vi "Run Test - Parameter Calculation (SubVI).vi"(6 "Tab Control":T2, 7 "DS in":T3 {"M Event" items=["Stop", "Running", "PID", "Up Limit", "Down Limit", "Load Limit"]; "Test Type" items=["Please Select", "Triaxial Shear", "Triaxial UU", "Shearbox", "Permeability", "Consolidation (Stepped Loading)/Swelling", "Saturation (Incremental)", "User Defined", "UCT", "Isotropic Consolidation", "Swelling Pressure"]; "Data"."Test Type" items=["Please Select", "Triaxial Shear", "Triaxial UU", "Shearbox", "Permeability", "Consolidation (Stepped Loading)/Swelling", "Saturation (Incremental)", "User Defined", "UCT", "Isotropic Consolidation", "Swelling Pressure"]}, 8 "error in (no error)":errorcluster, 9 "Decimal In":u8[](array[numeric]), 10 "Log Data In":string[](array[string]), 11 "Sensor Data In":sgl[](array[numeric])) -> (0 "error out":errorcluster, 3 "output cluster":T1, 5 "DS out":T3 {"M Event" items=["Stop", "Running", "PID", "Up Limit", "Down Limit", "Load Limit"]; "Test Type" items=["Please Select", "Triaxial Shear", "Triaxial UU", "Shearbox", "Permeability", "Consolidation (Stepped Loading)/Swelling", "Saturation (Incremental)", "User Defined", "UCT", "Isotropic Consolidation", "Swelling Pressure"]; "Data"."Test Type" items=["Please Select", "Triaxial Shear", "Triaxial UU", "Shearbox", "Permeability", "Consolidation (Stepped Loading)/Swelling", "Saturation (Incremental)", "User Defined", "UCT", "Isotropic Consolidation", "Swelling Pressure"]})   [LabVIEW 2019]
uses:
  Controls/RunTest - Data Structure.ctl
  Controls/Test Panel - Data Structure.ctl
  Controls/Station - Test Type.ctl
  <vilib>/Utility/miscctls.llb/LVRowAndColumnTypeDef.ctl
  Controls/RunTest - Calculate Data.ctl
  <vilib>/httpClient/ClientHandle.ctl
  Controls/RunTest - Start Condition.ctl
  Controls/RunTest - Stop Condition.ctl
  Controls/UDP - Event.ctl
  Controls/RunTest - Tab Test Type.ctl
  <vilib>/httpClient/LabVIEWHTTPClient.lvlib
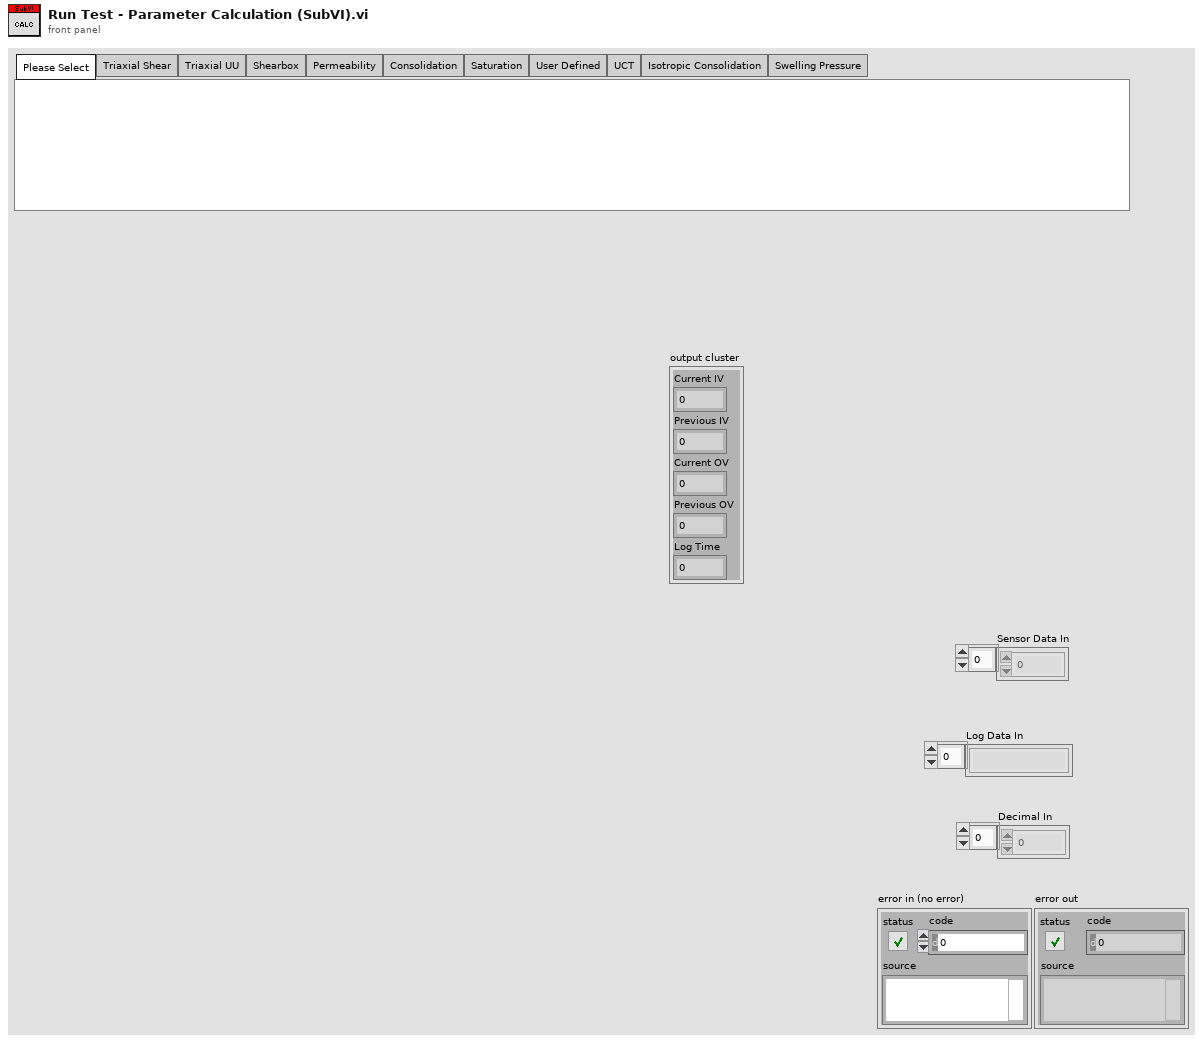
[diagram p1: front panel]
types:
  T1 = cluster{"Current IV":dbl, "Previous IV":dbl, "Current OV":dbl, "Previous OV":dbl, "Log Time":dbl}
  T2 = typedef "RunTest - Tab Test Type.ctl" = enum32{"Please Select", "Triaxial Shear", "Triaxial UU", "Shearbox", "Permeability", "Consolidation", "Saturation", "User Defined", "UCT", "Isotropic Consolidation", "Swelling Pressure"}
  T3 = typedef "RunTest - Data Structure.ctl" = cluster{"Test Plan":string[], "PlanRow":i32, "Device Name":string[], "Timeout":i32, "Start?":bool, "Pause?":bool, "IP Address":string[], "LogRow":i32, "Logtype":u16, "Log Elapse":sgl, "Data":T4, "Stop log?":bool, "tdms":refnum<k34>, "Sensor Data":sgl[], "Start time":timestamp, "Prev Log Elapse":u32, "Plot":u16, "X-Axis":u16[], "Y-Axis":u16[], "XY":cluster{"X":dbl, "Y":dbl}[][], "End Stage?":bool, "1run":bool, "Condition":u16[], "Start Con":bool, "Log Con":bool, "Stop Con":bool, "Start Elapse":dbl, "Start Load":dbl, "Motor":i32, "StartRow":i32, "number log":i32, "Dir":bool, "Start time test":timestamp, "Auto":bool, "Check return?":bool, "Inv":cluster{"M":i32[], "Bool":bool[]}, "tdms temp":refnum<k34>, "Zero?":bool, "Plot Timer":dbl, "1st Run":bool, "TDMS Path":path, "MaxLoad":dbl, "Log Timer":sgl[], "Test Type":T5, "Log Sensor":string[], "Save?":bool, "1st Log":bool, "Y-Axis 2":u16[], "On Y-Axis 2":bool, "Decimal":u8[], "Init":cluster{"PWP TS":sgl, "Load TS":sgl, "Volume TS":sgl, "Disp TS":sgl, "CP":sgl, "Vol In":sgl, "Vol Out":sgl, "Load UCT":sgl, "Disp UCT":sgl, "PWP Sat":sgl, "CP Sat":sgl, "Volume IsoCons":sgl, "PWP IsoCons":sgl, "PWP TUU":sgl, "Load TUU":sgl, "Volume TUU":sgl, "Disp TUU":sgl, "Load Cons":sgl, "Disp Cons":sgl, "Volume Sat":sgl, "Vertical Load SB":sgl, "Vertical Disp SB":sgl, "H Disp SB":sgl, "H Load SB":sgl}, "Calc":T7, "Device Index":i32[], "Channel Index":i32[], "http ref":T8, "fileid":string, "Step Cons":cluster{"V Stress":sgl, "H Settlement":sgl}, "RunTest":bool, "Graph Last":i32, "Init?":bool, "Datalog":bool[], "Start":T9, "Stop":T10, "Running?":bool, "StartTime":dbl, "Log Prev Time":dbl, "KeyName":string[], "Test RunTime":dbl, "Log Prev Axial":dbl, "M Event":T11[], "Last Log":bool, "popup":bool, "PreStart UU":bool, "PreStart Sat":bool}
  T4 = typedef "Test Panel - Data Structure.ctl" = cluster{"Station":string, "Sample ID":string, "Job No":string, "Job Description":string, "Filename":string, "Test Type":T5, "Speciment No":string, "Depth":string, "Height":string, "Diameter/Length":string, "Weight":string, "Test Parameter":string, "Station[]":string[], "Edit Pos":T6, "Edit Pos Prev":T6, "Area":string, "Path":string}
  T5 = typedef "Station - Test Type.ctl" = u16
  T6 = typedef "LVRowAndColumnTypeDef.ctl" = cluster{"Row":i32, "Column":i32}
  T7 = typedef "RunTest - Calculate Data.ctl" = cluster{"TS":cluster{"Change PWP":sgl, "Change Vol":sgl, "Axial Load":sgl, "CiL":sgl, "Deviator":sgl, "Axial Strain":sgl, "MaxDeviator":sgl}, "TUU":cluster{"Change PWP":sgl, "Axial Load":sgl, "CiL":sgl, "Deviator":sgl, "Axial Strain":sgl, "MaxDeviator":sgl}, "Sat":cluster{"B Value":sgl, "PWP Diss":sgl, "CPP":sgl, "CV":sgl}, "Per":cluster{"Change Vol In":sgl, "Change Vol Out":sgl, "Mean Vol":sgl, "Gradient Pressure":sgl, "Outlet Flow":sgl, "Inlet Flow":sgl, "I X1":sgl, "I X2":sgl, "I Y1":sgl, "I Y2":sgl, "O X1":sgl, "O X2":sgl, "O Y1":sgl, "O Y2":sgl}, "Step Cons":cluster{"V Stress":sgl, "H Settlement":sgl, "Total H Settle":sgl, "Prev Total H":sgl}, "UCT":cluster{"ALC":sgl, "H Change":sgl, "Deviator":sgl, "Axial Strain":sgl, "V Stress":sgl, "MaxDeviator":sgl}, "ISO Cons":cluster{"CPP":sgl, "PWP Diss":sgl, "CV":sgl}, "SB":cluster{"Speci LenC":sgl, "Shear Strain":sgl, "H LC":sgl, "Normal Stress":sgl, "Shear Stress":sgl, "MaxShear":sgl}}
  T8 = typedef "LabVIEWHTTPClient.lvlib/ClientHandle.ctl" = refnum<k1>
  T9 = typedef "RunTest - Start Condition.ctl" = cluster{"Cons":cluster{"VS":dbl, "Delay":bool, "No Delay":dbl}, "Sat":cluster{"CP":dbl, "BP":dbl, "StartBP":bool, "Target CP":bool, "Target BP":bool}, "Iso":cluster{"Select":dbl, "BP":dbl, "IC2":dbl, "IC3":dbl, "IC4":dbl, ". IC6":bool, "IC6":dbl, "IC6-2":dbl, "Target":bool, "Time Cond":dbl, "Last PWP":dbl}, "TS":cluster{"SS":dbl, "Engage":bool, "ES":dbl, "LC":dbl, "PreStart":bool, "Trig SS":bool, "Drain":dbl}, "TUU":cluster{"SS":dbl, "Engage":bool, "ES":dbl, "LC":dbl, "PreStart":bool, "Trig SS":bool, "CP":dbl, "Delay Value":dbl, "Delay":bool, "CP PID":bool}, "UCT":cluster{"SS":dbl, "Engage":bool, "ES":dbl, "LC":dbl, "PreStart":bool, "Trig SS":bool}, "Enable?":bool, "SB":cluster{"SS":dbl, "Engage":bool, "ES":dbl, "LC":dbl, "PreStart":bool, "Trig SS":bool, "VS":dbl, "Delay Value":dbl, "Delay":bool, "VS PID":bool}, "Perm":cluster{"DP":dbl}}
  T10 = typedef "RunTest - Stop Condition.ctl" = cluster{"Cons":cluster{"Select":i32, "Disp":dbl, "Time":dbl, "Time2":dbl, "Disp 2":dbl, "Time Cond":dbl, "Last Disp":dbl, "Swell":bool}, "Sat":cluster{"Select":i32, "PP":dbl, "Time":dbl, "VC":dbl, "Time2":dbl, "Time Cond":dbl, "Last PP":dbl, ".B":bool, "B":dbl, "Last Vc":dbl, "Time Cond 2":dbl, "Time3":dbl, "Time Cond 3":dbl, "B Achieve":bool}, "Iso":cluster{"PP":dbl, "Time":dbl, "VC":dbl, "Time2":dbl, "Time Cond":dbl, "Last Vc":dbl, ".PP":bool, "Time Cond 2":dbl, "Select":i32}, "TS":cluster{"Axial":dbl, ".MaxDev":bool, "MaxDev Value":dbl, "Return":bool, "Reset":bool, "Prev Time":dbl, "PostStop Run":bool, "CP Stop":bool, "BP Stop":bool, "PostStop Trig":bool, "Reset Value":dbl, "BPTrig":bool, "CPTrig":bool, "VLCTrig":bool}, "TUU":cluster{"Axial":dbl, ".MaxDev":bool, "MaxDev Value":dbl, "Return":bool, "Reset":bool, "Prev Time":dbl, "PostStop Run":bool, "CP Stop":bool, "BP Stop":bool, "PostStop Trig":bool, "Reset Value":dbl, "BPTrig":bool, "CPTrig":bool, "VLCTrig":bool}, "UCT":cluster{"Axial":dbl, ".MaxDev":bool, "MaxDev Value":dbl, "Return":bool, "Reset":bool, "Prev Time":dbl, "PostStop Run":bool, "CP Stop":bool, "BP Stop":bool, "PostStop Trig":bool}, "Enable?":bool, "SB":cluster{"Shear":dbl, ".MaxShear":bool, "MaxShear Value":dbl, "Return":bool, "Reset":bool, "Prev Time":dbl, "PostStop Run":bool, "CP Stop":bool, "BP Stop":bool, "PostStop Trig":bool, "Reset Value":dbl, "BPTrig":bool, "CPTrig":bool, "VLCTrig":bool}, "Perm":cluster{"Max Time":bool, "Reset":bool, "PostStop Run":bool, "Ratio":bool, "Reset Value":dbl, "Time":dbl, "RatioTime":dbl, "RatioMore":dbl, "RatioLess":dbl, "Time Cond":dbl, "Time Cond 2":dbl, "Prev IF":dbl, "Prev OF":dbl, "PostStop Trig":bool, "BP Trig":bool, "DP Stop":bool, "BP Stop":bool, "CP Stop":bool, "CP Trig":bool}, "SP":cluster{".Max Time":bool, ".Time":bool, "Time":dbl, "MaxTime":dbl, "Time Cond":dbl, "Max Time Cond":dbl, "Stress":dbl}}
  T11 = typedef "UDP - Event.ctl" = u16
  T12 = cluster{"Current IV":dbl, "Previous IV":dbl, "Current OV":dbl, "Previous OV":dbl, "Log time":dbl}
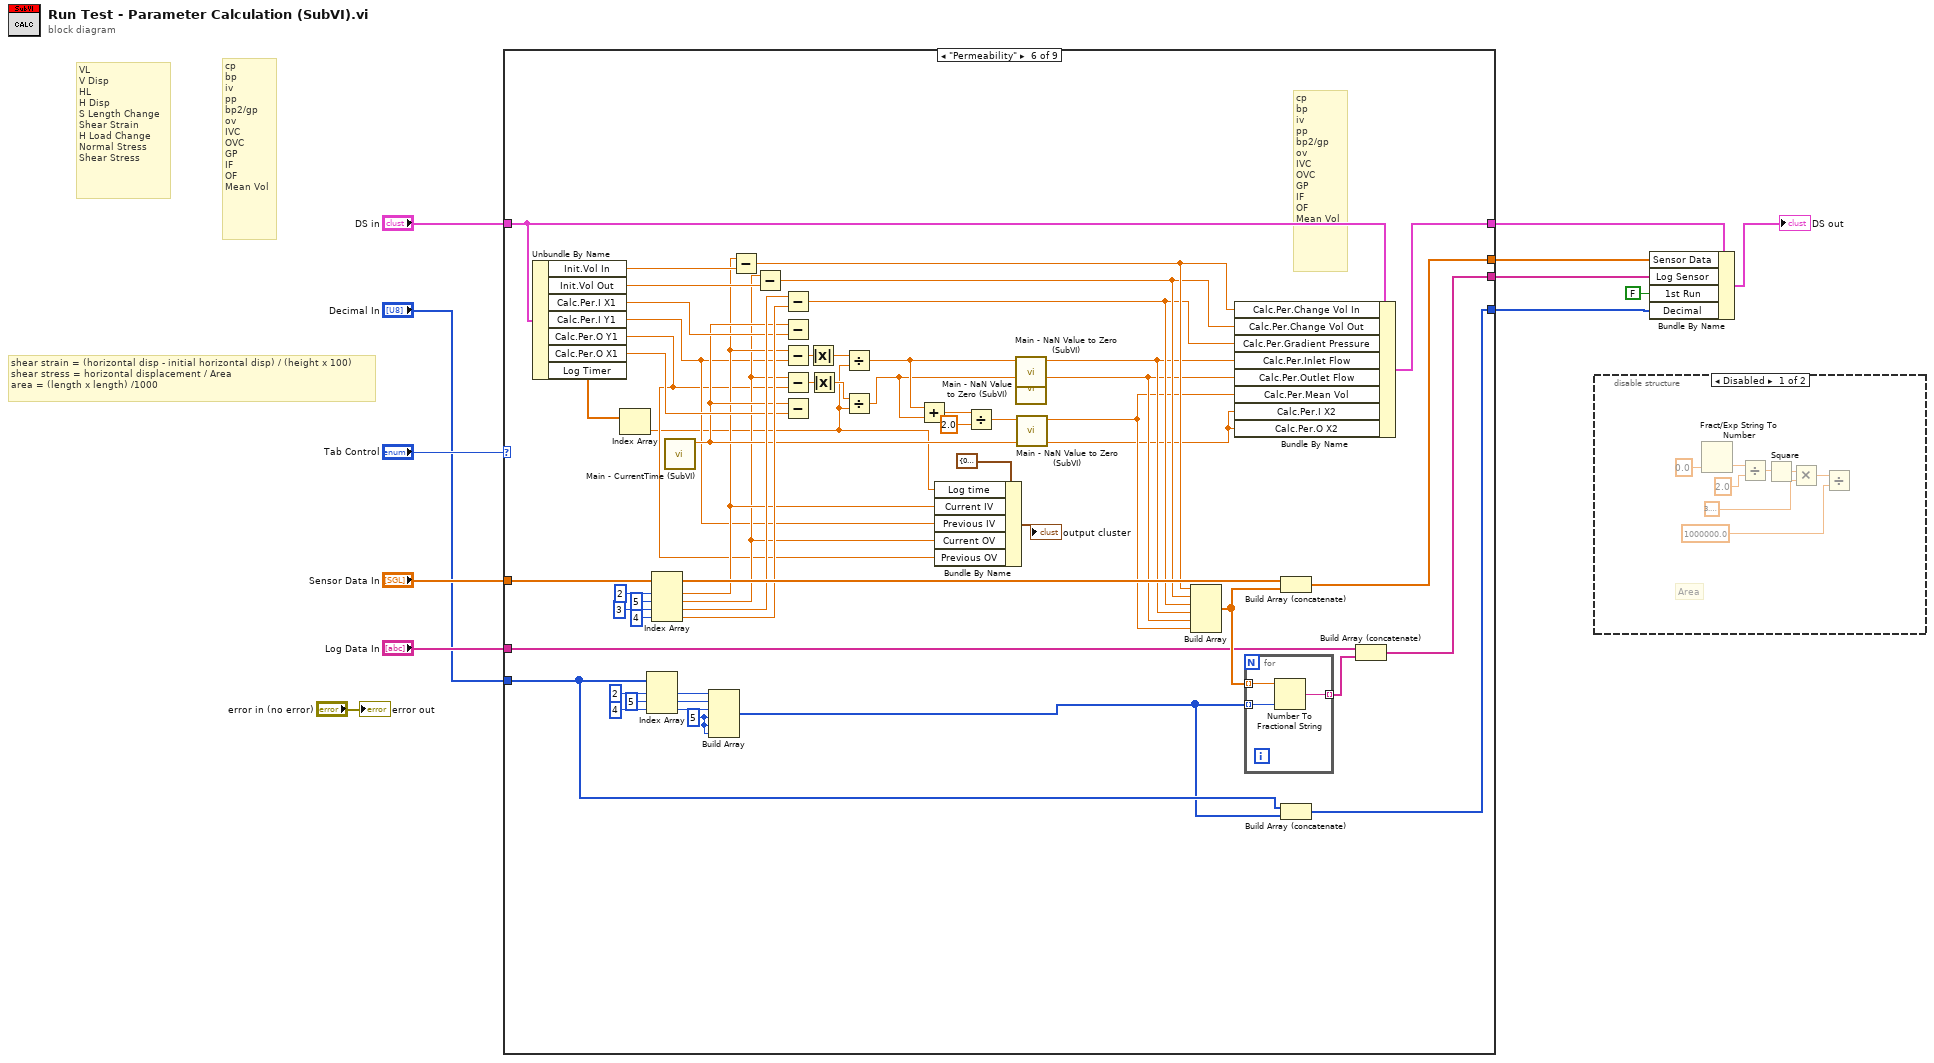
[diagram p0: block diagram]
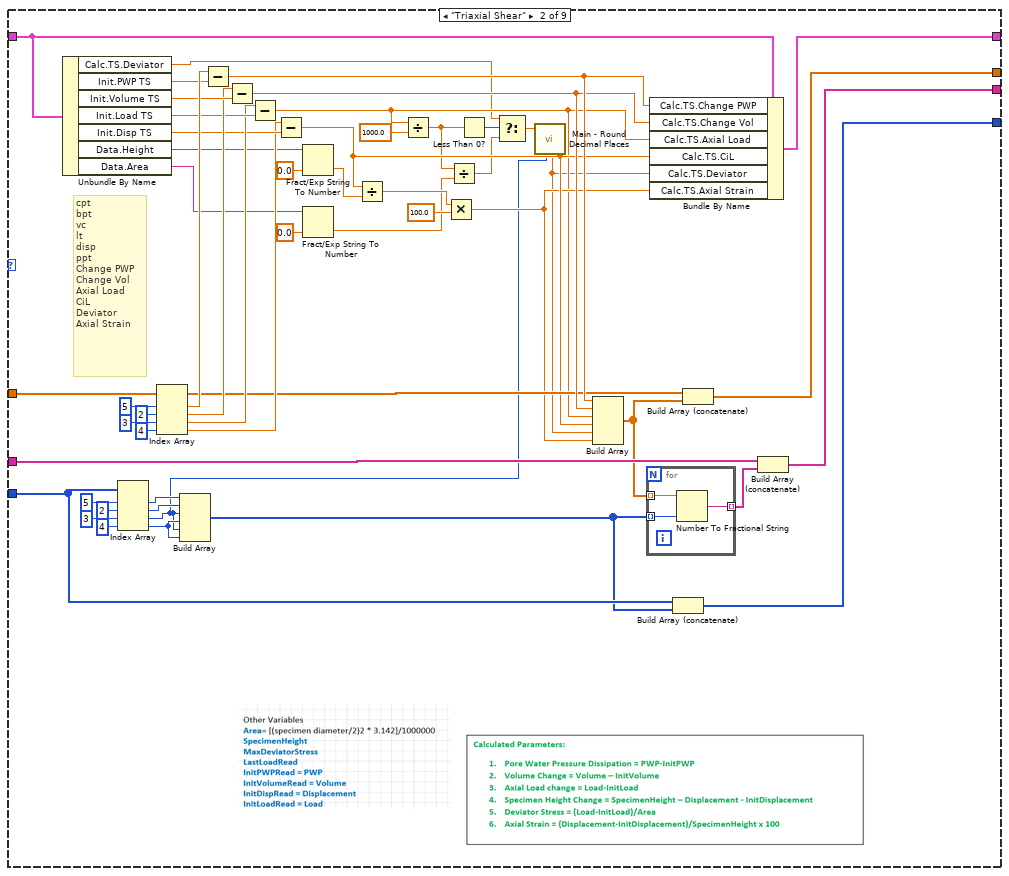
[diagram p4: hidden frame]
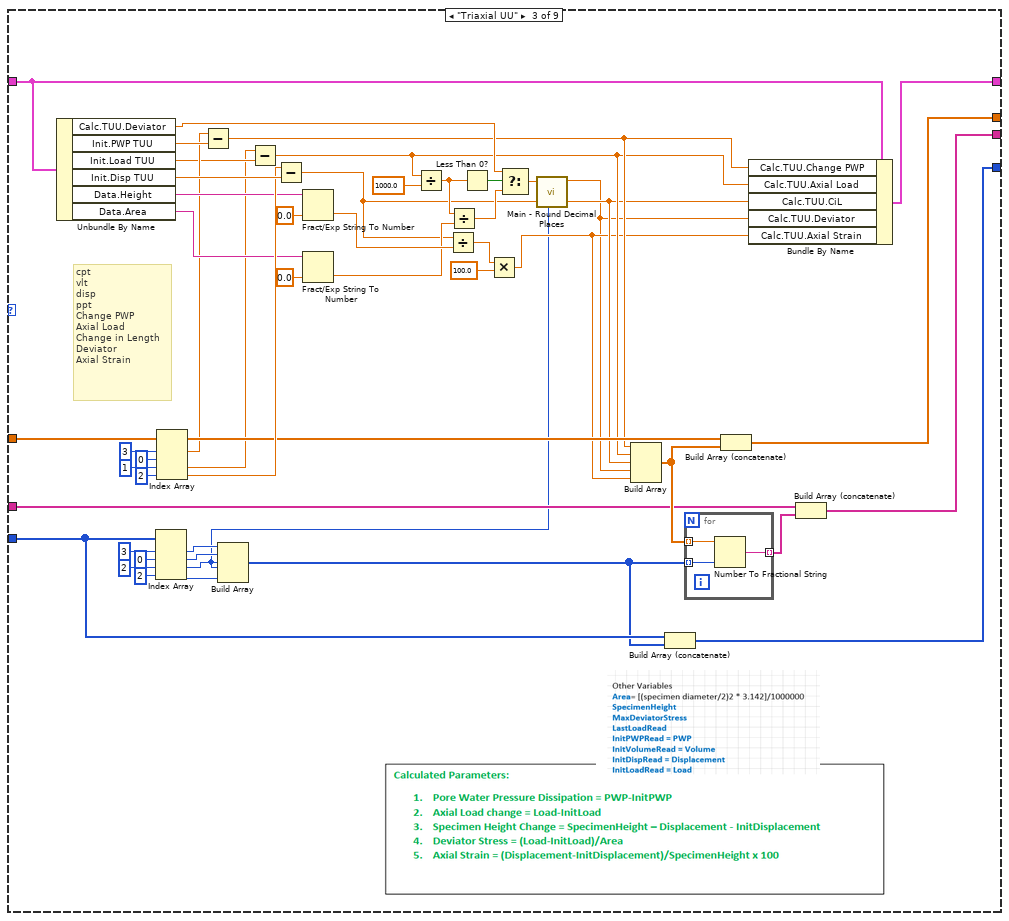
[diagram p5: hidden frame]
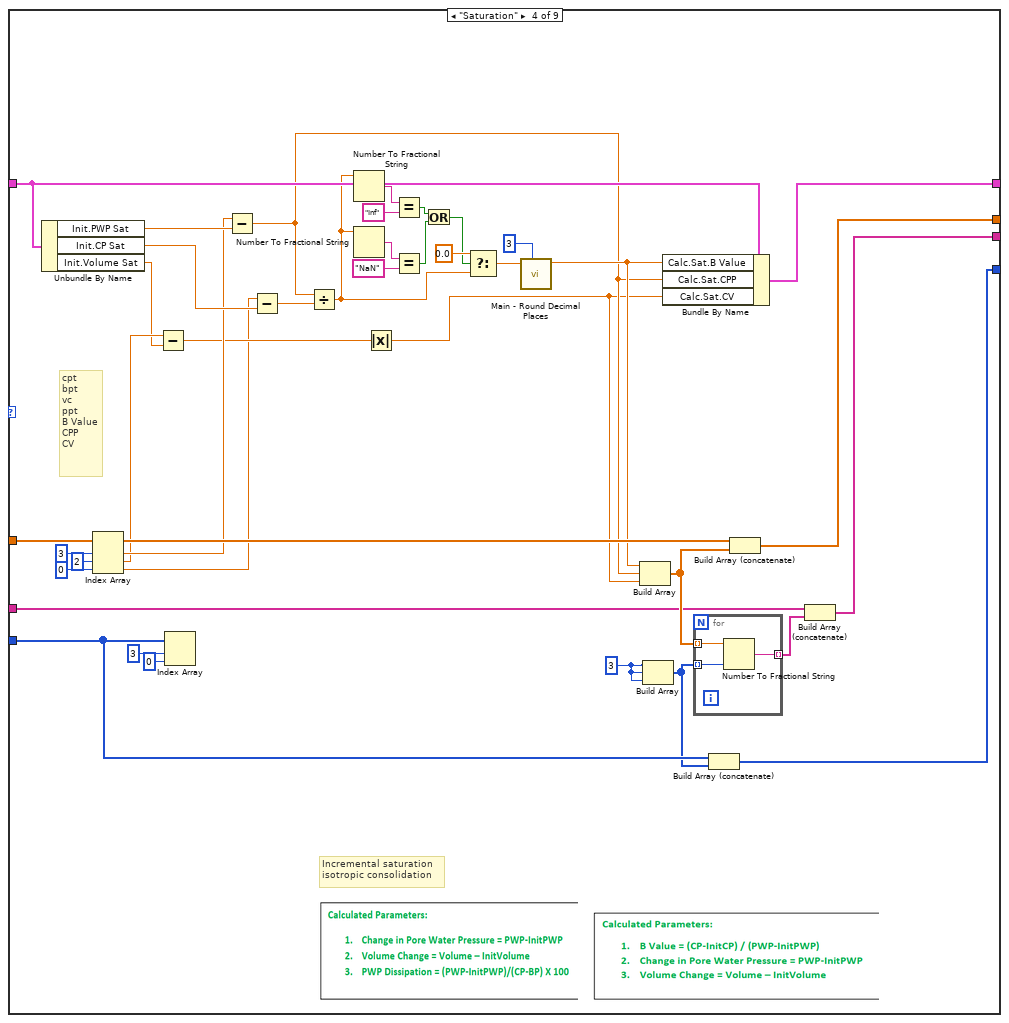
[diagram p6: hidden frame]
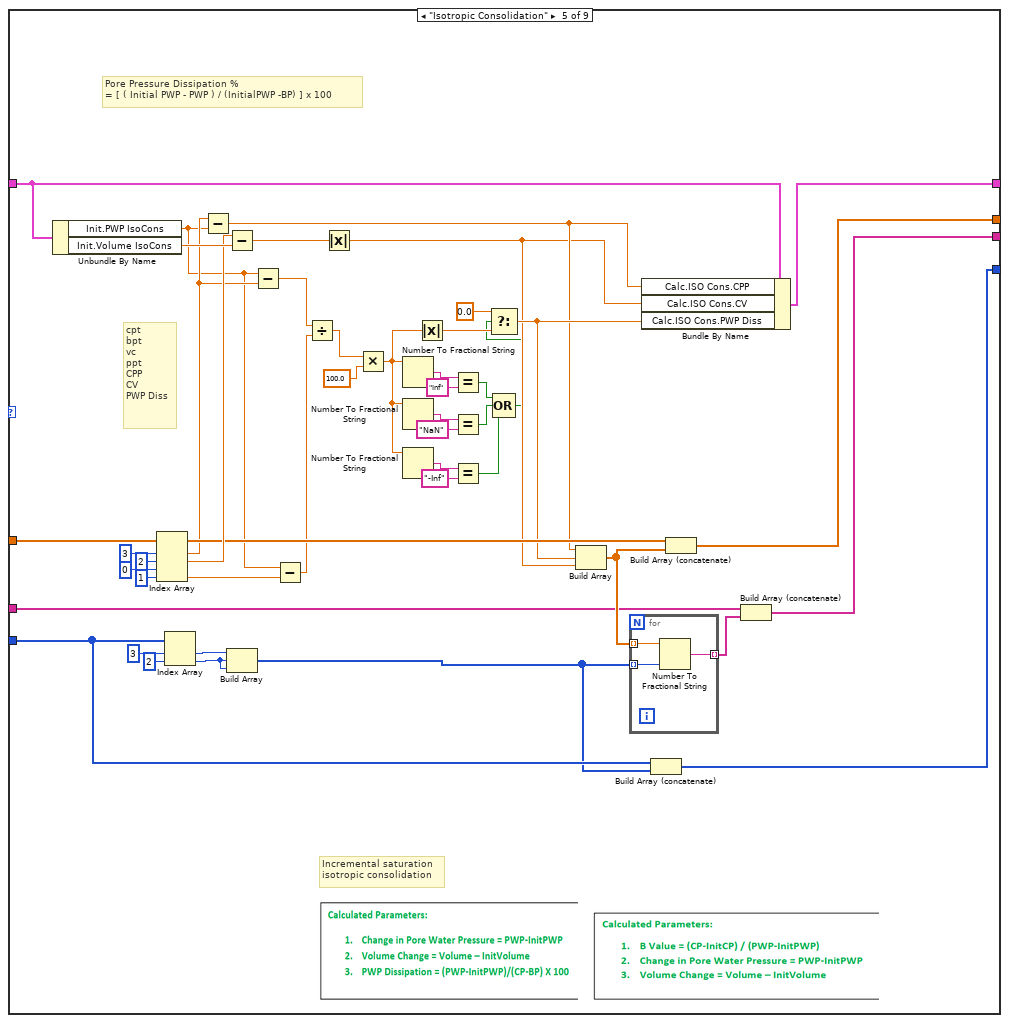
[diagram p7: hidden frame]
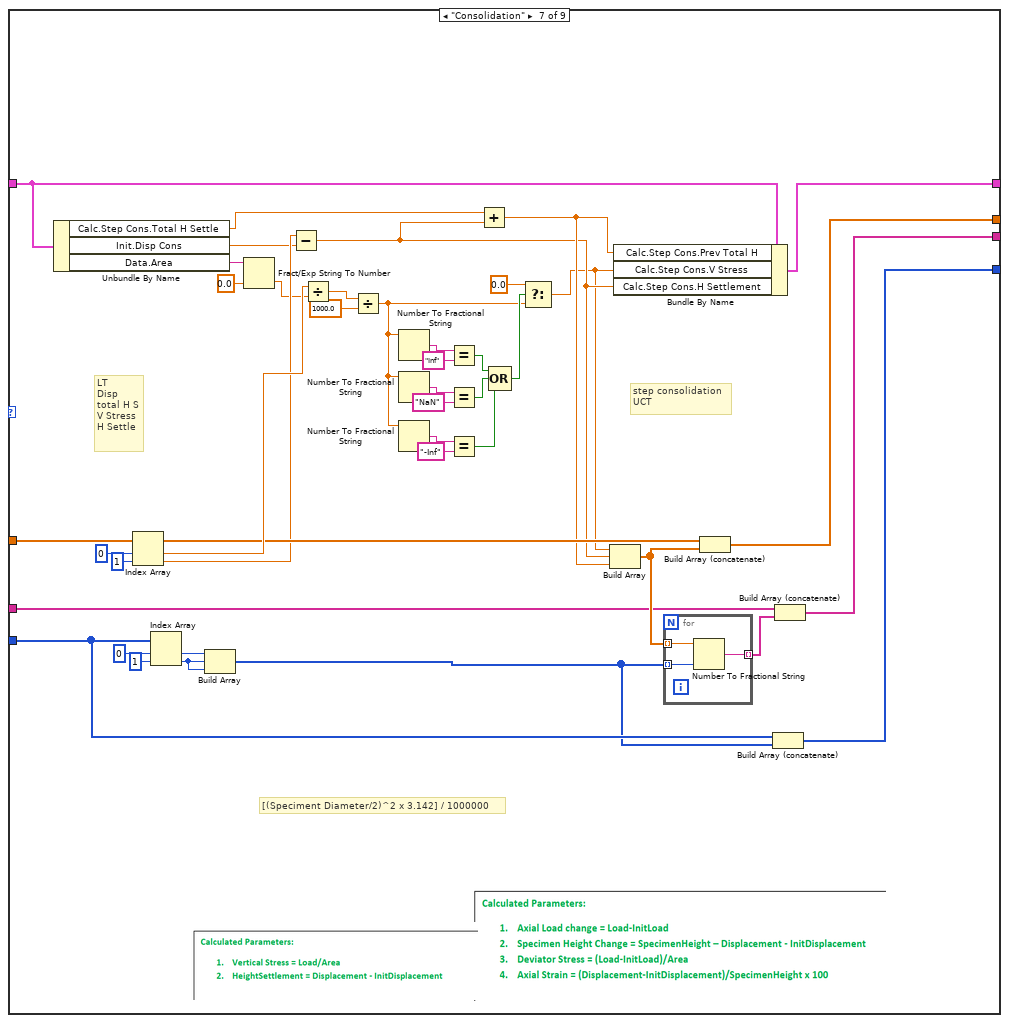
[diagram p8: hidden frame]
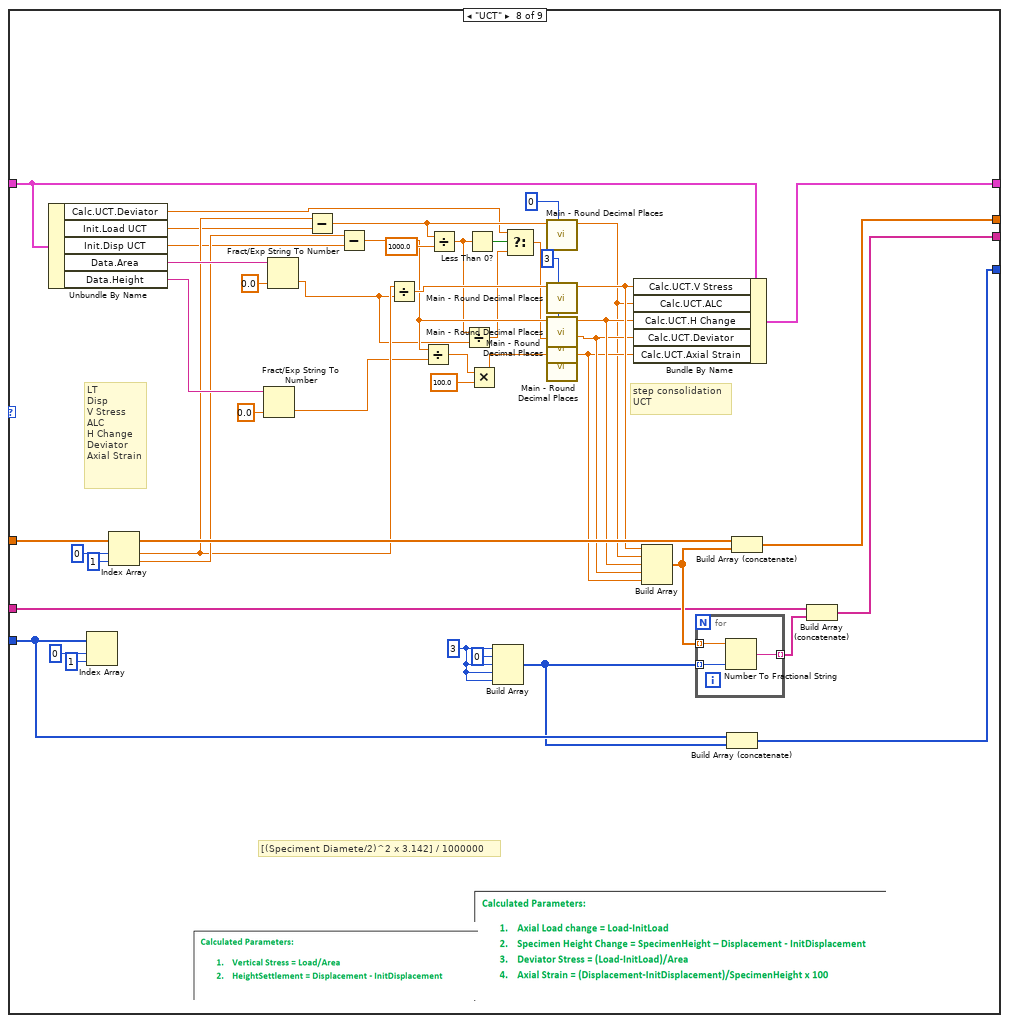
[diagram p9: hidden frame]
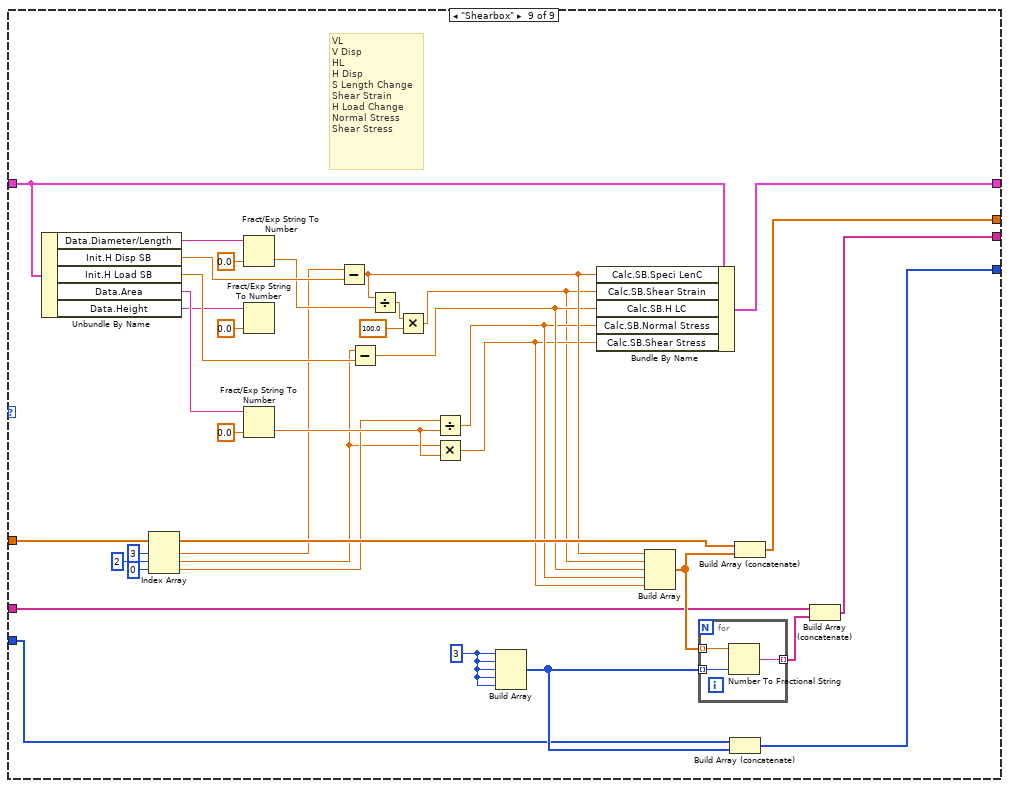
[diagram p10: hidden frame]
diagram:
  # "shear strain = (horizontal disp - initial horizontal disp) / (height x 100)\nshear stress = horizontal displacement / Area\narea = (length x length) /1000"
  # "cp\nbp\niv\npp\nbp2/gp\nov\nIVC\nOVC\nGP\nIF\nOF\nMean Vol"
  # "VL\nV Disp\nHL\nH Disp\nS Length Change\nShear Strain\nH Load Change\nNormal Stress\nShear Stress"
  n1 = case shown="\"Permeability\"" "Tab Control" {
    tunnel: "Sensor Data In" -> [w15 w38 w98 w151 w194 w252 w297 w342 w379]
    tunnel: [w16 w55 w112 w157 w202 w259 w305 w354 w390] -> w7
    tunnel: "DS in" -> [w16 w54 w111 w156 w201 w258 w304 w353 w389]
    tunnel: [w15 w37 w95 w150 w193 w251 w296 w341 w373] -> w5
    tunnel: "Log Data In" -> [w14 w46 w99 w152 w195 w253 w298 w343 w377]
    tunnel: "Decimal In" -> [w13 w27 w87 w124 w180 w247 w285 w321 w378]
    tunnel: [w14 w34 w96 w149 w192 w250 w295 w340 w372] -> w3
    tunnel: [w13 w25 w86 w122 w178 w245 w283 w319 w371] -> w1
    frame "Please Select", Default {
    }
    frame "Triaxial Shear" {
      # "cpt\nbpt\nvc\nlt\ndisp\nppt\nChange PWP\nChange Vol\nAxial Load\nCiL\nDeviator\nAxial Strain"
      n2 = Unbundle By Name(w54) -> ("Calc.TS.Deviator"=w20:sgl, "Init.PWP TS"=w65:sgl, "Init.Volume TS"=w63:sgl, "Init.Load TS"=w60:sgl, "Init.Disp TS"=w57:sgl, "Data.Height"=w53:string, "Data.Area"=w50:string)
      n3 = Index Array(array=w27, index #1=5 ("index"), index #2=2 ("index"), index #3=3 ("index"), index #4=4 ("index")) -> (element #1=w41:u8, element #2=w40:u8, element #3=w17:u8, element #4=w39:u8)
      n4 = Index Array(array=w38, index #1=5 ("index"), index #2=2 ("index"), index #3=3 ("index"), index #4=4 ("index")) -> (element #1=w66:sgl, element #2=w62:sgl, element #3=w59:sgl, element #4=w56:sgl)
      n5 = Build Array(w41, w40, w17, w39, w17, w39) -> (w26:u8[])
      n6 = Subtract(x=w66, y=w65) -> (x-y=w48:sgl)
      n7 = Subtract(x=w62, y=w63) -> (x-y=w47:sgl)
      n8 = Subtract(x=w59, y=w60) -> (x-y=w28:sgl)
      n9 = Subtract(x=w56, y=w57) -> (x-y=w33:sgl)
      n10 = Fract/Exp String To Number(string=w53, default (0 dbl)=sgl 0.0 ("default (0 DBL)")) -> (number=w32:sgl)  [unwired: 2 in, 1 out]
      n11 = Fract/Exp String To Number(string=w50, default (0 dbl)=sgl 0.0 ("default (0 DBL)")) -> (number=w24:sgl)  [unwired: 2 in, 1 out]
      n12 = Divide(x=w33, y=w32) -> (x/y=w31:sgl)
      n13 = Divide(x=w28, y=sgl 1000.0) -> (x/y=w22:sgl)
      n14 = Multiply(x=w31, y=sgl 100.0) -> (x*y=w30:sgl)
      n15 = Divide(x=w22, y=w24) -> (x/y=w21:sgl)
      n16 = Less Than 0?(x=w22) -> (x < 0?=w23:bool)
      n17 = Select(t=w20, s=w23, f=w21) -> (s? t:f=w19:sgl)
      n18 = call "Main - Round Decimal Places.vi"("DecimalPlaces"=w17, "Number to round"=w19) -> ("Rounded number"=w18:dbl)  [unwired: 9 in]
      n19 = Build Array(w48, w47, w28, w33, w18, w30) -> (w36:dbl[])
      n20 = for {
        tunnel: w36 -> [w70] mode=indexing
        tunnel: w26 -> [w69] mode=indexing
        tunnel: [w68] -> w35 mode=indexing
        n21 = Number To Fractional String(number=w70, precision (6)=w69) -> (F-format string=w68:string)  [unwired: 2 in]
      }
      n22 = Bundle By Name(cluster=w54, "Calc.TS.Change PWP"=w48, "Calc.TS.Change Vol"=w47, "Calc.TS.Axial Load"=w28, "Calc.TS.CiL"=w33, "Calc.TS.Deviator"=w18, "Calc.TS.Axial Strain"=w30) -> (w55:T3)
      n23 = Build Array (concatenate)(w27, w26) -> (w25:u8[])
      n24 = Build Array (concatenate)(w38, w36) -> (w37:dbl[])
      n25 = Build Array (concatenate)(w46, w35) -> (w34:string[])
    }
    frame "Triaxial UU" {
      # "cpt\nvlt\ndisp\nppt\nChange PWP\nAxial Load\nChange in Length\nDeviator\nAxial Strain"
      n26 = Unbundle By Name(w111) -> ("Calc.TUU.Deviator"=w81:sgl, "Init.PWP TUU"=w91:sgl, "Init.Load TUU"=w89:sgl, "Init.Disp TUU"=w114:sgl, "Data.Height"=w110:string, "Data.Area"=w107:string)
      n27 = Index Array(array=w87, index #1=3 ("index"), index #2=0 ("index"), index #3=2 ("index"), index #4=2 ("index")) -> (element #1=w80:u8, element #2=w72:u8, element #3=w71:u8, element #4=w97:u8)
      n28 = Index Array(array=w98, index #1=3 ("index"), index #2=0 ("index"), index #3=1 ("index"), index #4=2 ("index")) -> (element #1=w90:sgl, element #3=w88:sgl, element #4=w113:sgl)  [unwired: 1 out]
      n29 = Subtract(x=w90, y=w91) -> (x-y=w78:sgl)
      n30 = Build Array(w80, w72, w71, w71, w97) -> (w79:u8[])
      n31 = Subtract(x=w88, y=w89) -> (x-y=w77:sgl)
      n32 = Subtract(x=w113, y=w114) -> (x-y=w76:sgl)
      n33 = Fract/Exp String To Number(string=w110, default (0 dbl)=sgl 0.0 ("default (0 DBL)")) -> (number=w94:sgl)  [unwired: 2 in, 1 out]
      n34 = Fract/Exp String To Number(string=w107, default (0 dbl)=sgl 0.0 ("default (0 DBL)")) -> (number=w85:sgl)  [unwired: 2 in, 1 out]
      n35 = Divide(x=w77, y=sgl 1000.0) -> (x/y=w84:sgl)
      n36 = Divide(x=w76, y=w94) -> (x/y=w93:sgl)
      n37 = Divide(x=w84, y=w85) -> (x/y=w82:sgl)
      n38 = Less Than 0?(x=w84) -> (x < 0?=w83:bool)
      n39 = Multiply(x=w93, y=sgl 100.0) -> (x*y=w75:sgl)
      n40 = Select(t=w81, s=w83, f=w82) -> (s? t:f=w74:sgl)
      n41 = call "Main - Round Decimal Places.vi"("DecimalPlaces"=w71, "Number to round"=w74) -> ("Rounded number"=w73:dbl)  [unwired: 9 in]
      n42 = Build Array(w78, w77, w76, w73, w75) -> (w101:dbl[])
      n43 = Build Array (concatenate)(w87, w79) -> (w86:u8[])
      n44 = for {
        tunnel: w101 -> [w121] mode=indexing
        tunnel: w79 -> [w120] mode=indexing
        tunnel: [w119] -> w100 mode=indexing
        n45 = Number To Fractional String(number=w121, precision (6)=w120) -> (F-format string=w119:string)  [unwired: 2 in]
      }
      n46 = Build Array (concatenate)(w98, w101) -> (w95:dbl[])
      n47 = Bundle By Name(cluster=w111, "Calc.TUU.Change PWP"=w78, "Calc.TUU.Axial Load"=w77, "Calc.TUU.CiL"=w76, "Calc.TUU.Deviator"=w73, "Calc.TUU.Axial Strain"=w75) -> (w112:T3)
      n48 = Build Array (concatenate)(w99, w100) -> (w96:string[])
    }
    frame "Saturation" {
      w127 = u8 3 ("index")
      # "Incremental saturation\nisotropic consolidation"
      # "cpt\nbpt\nvc\nppt\nB Value\nCPP\nCV"
      n49 = Unbundle By Name(w156) -> ("Init.PWP Sat"=w133:sgl, "Init.CP Sat"=w136:sgl, "Init.Volume Sat"=w130:sgl)
      n50 = Index Array(array=w151, index #1=3 ("index"), index #2=2 ("index"), index #3=0 ("index")) -> (element #1=w132:sgl, element #2=w131:sgl, element #3=w128:sgl)
      n51 = Subtract(x=w131, y=w130) -> (x-y=w129:sgl)
      n52 = Index Array(array=w124, index #1=3 ("index"), index #2=0 ("index")) -> ()  [unwired: 2 out]
      n53 = Subtract(x=w132, y=w133) -> (x-y=w126:sgl)
      n54 = Subtract(x=w128, y=w136) -> (x-y=w135:sgl)
      n55 = Divide(x=w126, y=w135) -> (x/y=w134:sgl)
      n56 = Number To Fractional String(number=w134) -> (F-format string=w140:string)  [unwired: 3 in]
      n57 = Number To Fractional String(number=w134) -> (F-format string=w147:string)  [unwired: 3 in]
      n58 = Absolute Value(x=w129) -> (abs(x)=w125:sgl)
      n59 = Equal?(x=w140, y="Inf") -> (x = y?=w139:bool)
      n60 = Equal?(x=w147, y="NaN") -> (x = y?=w138:bool)
      n61 = Or(x=w139, y=w138) -> (x .or. y?=w137:bool)
      n62 = Select(t=sgl 0.0, s=w137, f=w134) -> (s? t:f=w145:sgl)
      n63 = call "Main - Round Decimal Places.vi"("DecimalPlaces"=u8 3, "Number to round"=w145) -> ("Rounded number"=w144:dbl)  [unwired: 9 in]
      n64 = Build Array(w144, w126, w125) -> (w154:dbl[])
      n65 = Build Array(w127, w127, w127) -> (w123:u8[])
      n66 = Bundle By Name(cluster=w156, "Calc.Sat.B Value"=w144, "Calc.Sat.CPP"=w126, "Calc.Sat.CV"=w125) -> (w157:T3)
      n67 = for {
        tunnel: w154 -> [w163] mode=indexing
        tunnel: w123 -> [w162] mode=indexing
        tunnel: [w161] -> w153 mode=indexing
        n68 = Number To Fractional String(number=w163, precision (6)=w162) -> (F-format string=w161:string)  [unwired: 2 in]
      }
      n69 = Build Array (concatenate)(w124, w123) -> (w122:u8[])
      n70 = Build Array (concatenate)(w151, w154) -> (w150:dbl[])
      n71 = Build Array (concatenate)(w152, w153) -> (w149:string[])
    }
    frame "Isotropic Consolidation" {
      # "Pore Pressure Dissipation %\n= [ ( Initial PWP - PWP ) / (InitialPWP -BP) ] x 100"
      # "Incremental saturation\nisotropic consolidation"
      # "cpt\nbpt\nvc\nppt\nCPP\nCV\nPWP Diss"
      n72 = Unbundle By Name(w201) -> ("Init.PWP IsoCons"=w175:sgl, "Init.Volume IsoCons"=w206:sgl)
      n73 = Index Array(array=w194, index #1=3 ("index"), index #2=2 ("index"), index #3=0 ("index"), index #4=1 ("index")) -> (element #1=w177:sgl, element #2=w205:sgl, element #4=w174:sgl)  [unwired: 1 out]
      n74 = Index Array(array=w180, index #1=3 ("index"), index #2=2 ("index")) -> (element #1=w191:u8, element #2=w181:u8)
      n75 = Subtract(x=w177, y=w175) -> (x-y=w184:sgl)
      n76 = Subtract(x=w205, y=w206) -> (x-y=w190:sgl)
      n77 = Build Array(w191, w181, w181) -> (w179:u8[])
      n78 = Subtract(x=w175, y=w177) -> (x-y=w176:sgl)
      n79 = Subtract(x=w175, y=w174) -> (x-y=w183:sgl)
      n80 = Divide(x=w176, y=w183) -> (x/y=w185:sgl)
      n81 = Absolute Value(x=w190) -> (abs(x)=w182:sgl)
      n82 = Multiply(x=w185, y=sgl 100.0) -> (x*y=w168:sgl)
      n83 = Number To Fractional String(number=w168) -> (F-format string=w189:string)  [unwired: 3 in]
      n84 = Number To Fractional String(number=w168) -> (F-format string=w171:string)  [unwired: 3 in]
      n85 = Number To Fractional String(number=w168) -> (F-format string=w170:string)  [unwired: 3 in]
      n86 = Absolute Value(x=w168) -> (abs(x)=w173:sgl)
      n87 = Equal?(x=w189, y="Inf") -> (x = y?=w167:bool)
      n88 = Equal?(x=w171, y="NaN") -> (x = y?=w166:bool)
      n89 = Equal?(x=w170, y="-Inf") -> (x = y?=w165:bool)
      n90 = Compound Arithmetic op=OR(w167, w166, w165) -> (w164:bool)
      n91 = Select(t=sgl 0.0, s=w164, f=w173) -> (s? t:f=w187:sgl)
      n92 = Build Array(w184, w187, w182) -> (w197:sgl[])
      n93 = for {
        tunnel: w197 -> [w211] mode=indexing
        tunnel: w179 -> [w210] mode=indexing
        tunnel: [w209] -> w196 mode=indexing
        n94 = Number To Fractional String(number=w211, precision (6)=w210) -> (F-format string=w209:string)  [unwired: 2 in]
      }
      n95 = Bundle By Name(cluster=w201, "Calc.ISO Cons.CPP"=w184, "Calc.ISO Cons.CV"=w182, "Calc.ISO Cons.PWP Diss"=w187) -> (w202:T3)
      n96 = Build Array (concatenate)(w180, w179) -> (w178:u8[])
      n97 = Build Array (concatenate)(w194, w197) -> (w193:sgl[])
      n98 = Build Array (concatenate)(w195, w196) -> (w192:string[])
    }
    frame "Permeability" {
      w212 = u8 5 ("element")
      # "cp\nbp\niv\npp\nbp2/gp\nov\nIVC\nOVC\nGP\nIF\nOF\nMean Vol"
      n99 = Unbundle By Name(w258) -> ("Init.Vol In"=w262:sgl, "Init.Vol Out"=w260:sgl, "Calc.Per.I X1"=w240:sgl, "Calc.Per.I Y1"=w217:sgl, "Calc.Per.O Y1"=w216:sgl, "Calc.Per.O X1"=w238:sgl, "Log Timer"=w221:sgl[])
      n100 = Index Array(array=w221) -> (element=w214:sgl)  [unwired: 1 in]
      n101 = Index Array(array=w247, index #1=2 ("index"), index #2=5 ("index"), index #3=4 ("index")) -> (element #1=w231:u8, element #2=w213:u8, element #3=w232:u8)
      n102 = Index Array(array=w252, index #1=2 ("index"), index #2=5 ("index"), index #3=3 ("index"), index #4=4 ("index")) -> (element #1=w219:sgl, element #2=w218:sgl, element #3=w242:sgl, element #4=w241:sgl)
      n103 = call "Main - CurrentTime (SubVI).vi"() -> ("Seconds"=w222:dbl)  [unwired: 10 in, 1 out]
      n104 = Build Array(w231, w213, w232, w212, w212, w212) -> (w246:u8[])
      n105 = Subtract(x=w219, y=w262) -> (x-y=w249:sgl)
      n106 = Subtract(x=w218, y=w260) -> (x-y=w248:sgl)
      n107 = Subtract(x=w242, y=w241) -> (x-y=w234:sgl)
      n108 = Subtract(x=w222, y=w240) -> ()  [unwired: 1 out]
      n109 = Subtract(x=w219, y=w217) -> (x-y=w239:sgl)
      n110 = Subtract(x=w218, y=w216) -> (x-y=w237:sgl)
      n111 = Subtract(x=w222, y=w238) -> ()  [unwired: 1 out]
      n112 = Absolute Value(x=w239) -> (abs(x)=w223:sgl)
      n113 = Absolute Value(x=w237) -> (abs(x)=w224:sgl)
      n114 = Divide(x=w223, y=w214) -> (x/y=w230:sgl)
      n115 = Divide(x=w224, y=w214) -> (x/y=w228:sgl)
      n116 = Add(x=w230, y=w228) -> (x+y=w236:sgl)
      n117 = Bundle By Name(cluster=T12 {"Current IV"=0.0, "Previous IV"=0.0, "Current OV"=0.0, "Previous OV"=0.0, "Log time"=0.0}, "Log time"=w214, "Current IV"=w219, "Previous IV"=w217, "Current OV"=w218, "Previous OV"=w216) -> (→"output cluster":T12)
      n118 = Divide(x=w236, y=sgl 2.0) -> (x/y=w226:sgl)
      n119 = call "Main - NaN Value to Zero (SubVI).vi"("Input"=w230) -> ("Output"=w229:sgl)  [unwired: 10 in]
      n120 = call "Main - NaN Value to Zero (SubVI).vi"("Input"=w228) -> ("Output"=w227:sgl)  [unwired: 10 in]
      n121 = call "Main - NaN Value to Zero (SubVI).vi"("Input"=w226) -> ("Output"=w225:sgl)  [unwired: 10 in]
      n122 = Build Array(w249, w248, w234, w229, w227, w225) -> (w255:sgl[])
      n123 = Bundle By Name(cluster=w258, "Calc.Per.Change Vol In"=w249, "Calc.Per.Change Vol Out"=w248, "Calc.Per.Gradient Pressure"=w234, "Calc.Per.Inlet Flow"=w229, "Calc.Per.Outlet Flow"=w227, "Calc.Per.Mean Vol"=w225, "Calc.Per.I X2"=w222, "Calc.Per.O X2"=w222) -> (w259:T3)
      n124 = for {
        tunnel: w255 -> [w266] mode=indexing
        tunnel: w246 -> [w265] mode=indexing
        tunnel: [w264] -> w254 mode=indexing
        n125 = Number To Fractional String(number=w266, precision (6)=w265) -> (F-format string=w264:string)  [unwired: 2 in]
      }
      n126 = Build Array (concatenate)(w252, w255) -> (w251:sgl[])
      n127 = Build Array (concatenate)(w247, w246) -> (w245:u8[])
      n128 = Build Array (concatenate)(w253, w254) -> (w250:string[])
    }
    frame "Consolidation" {
      # "[(Speciment Diameter/2)^2 x 3.142] / 1000000"
      # "LT\nDisp\ntotal H S\nV Stress\nH Settle"
      # "step consolidation\nUCT"
      n129 = Unbundle By Name(w304) -> ("Calc.Step Cons.Total H Settle"=w289:sgl, "Init.Disp Cons"=w290:sgl, "Data.Area"=w281:string)
      n130 = Index Array(array=w297, index #1=0 ("index"), index #2=1 ("index")) -> (element #1=w303:sgl, element #2=w291:sgl)
      n131 = Index Array(array=w285, index #1=0 ("index"), index #2=1 ("index")) -> (element #1=w294:u8, element #2=w288:u8)
      n132 = Build Array(w294, w288, w288) -> (w284:u8[])
      n133 = Fract/Exp String To Number(string=w281, default (0 dbl)=sgl 0.0 ("default (0 DBL)")) -> (number=w280:sgl)  [unwired: 2 in, 1 out]
      n134 = Subtract(x=w291, y=w290) -> (x-y=w286:sgl)
      n135 = Divide(x=w303, y=w280) -> (x/y=w292:sgl)
      n136 = Divide(x=w292, y=1000.0) -> (x/y=w268:dbl)
      n137 = Number To Fractional String(number=w268) -> (F-format string=w279:string)  [unwired: 3 in]
      n138 = Number To Fractional String(number=w268) -> (F-format string=w275:string)  [unwired: 3 in]
      n139 = Number To Fractional String(number=w268) -> (F-format string=w274:string)  [unwired: 3 in]
      n140 = Equal?(x=w279, y="Inf") -> (x = y?=w272:bool)
      n141 = Equal?(x=w275, y="NaN") -> (x = y?=w271:bool)
      n142 = Equal?(x=w274, y="-Inf") -> (x = y?=w270:bool)
      n143 = Add(x=w289, y=w286) -> (x+y=w287:sgl)
      n144 = Compound Arithmetic op=OR(w272, w271, w270) -> (w269:bool)
      n145 = Select(t=sgl 0.0, s=w269, f=w268) -> (s? t:f=w267:dbl)
      n146 = Build Array(w267, w286, w287) -> (w300:dbl[])
      n147 = Bundle By Name(cluster=w304, "Calc.Step Cons.Prev Total H"=w287, "Calc.Step Cons.V Stress"=w267, "Calc.Step Cons.H Settlement"=w286) -> (w305:T3)
      n148 = for {
        tunnel: w300 -> [w310] mode=indexing
        tunnel: w284 -> [w309] mode=indexing
        tunnel: [w308] -> w299 mode=indexing
        n149 = Number To Fractional String(number=w310, precision (6)=w309) -> (F-format string=w308:string)  [unwired: 2 in]
      }
      n150 = Build Array (concatenate)(w297, w300) -> (w296:dbl[])
      n151 = Build Array (concatenate)(w285, w284) -> (w283:u8[])
      n152 = Build Array (concatenate)(w298, w299) -> (w295:string[])
    }
    frame "UCT" {
      w312 = u8 3 ("DecimalPlaces")
      w332 = u8 3 ("element")
      # "[(Speciment Diamete/2)^2 x 3.142] / 1000000"
      # "LT\nDisp\nV Stress\nALC\nH Change\nDeviator\nAxial Strain"
      # "step consolidation\nUCT"
      n153 = Unbundle By Name(w353) -> ("Calc.UCT.Deviator"=w313:sgl, "Init.Load UCT"=w336:sgl, "Init.Disp UCT"=w337:sgl, "Data.Area"=w351:string, "Data.Height"=w349:string)
      n154 = Index Array(array=w321, index #1=0 ("index"), index #2=1 ("index")) -> ()  [unwired: 2 out]
      n155 = Index Array(array=w342, index #1=0 ("index"), index #2=1 ("index")) -> (element #1=w338:sgl, element #2=w339:sgl)
      n156 = Fract/Exp String To Number(string=w349, default (0 dbl)=sgl 0.0 ("default (0 DBL)")) -> (number=w335:sgl)  [unwired: 2 in, 1 out]
      n157 = Fract/Exp String To Number(string=w351, default (0 dbl)=sgl 0.0 ("default (0 DBL)")) -> (number=w318:sgl)  [unwired: 2 in, 1 out]
      n158 = Subtract(x=w338, y=w336) -> (x-y=w324:sgl)
      n159 = Subtract(x=w339, y=w337) -> (x-y=w329:sgl)
      n160 = Divide(x=w338, y=w318) -> (x/y=w331:sgl)
      n161 = Divide(x=w329, y=w335) -> (x/y=w334:sgl)
      n162 = Divide(x=w324, y=sgl 1000.0) -> (x/y=w316:sgl)
      n163 = Divide(x=w316, y=w318) -> (x/y=w315:sgl)
      n164 = Less Than 0?(x=w316) -> (x < 0?=w317:bool)
      n165 = Multiply(x=w334, y=sgl 100.0) -> (x*y=w326:sgl)
      n166 = Build Array(w332, u8 0 ("element"), w332, w332, w332) -> (w320:u8[])
      n167 = Select(t=w313, s=w317, f=w315) -> (s? t:f=w314:sgl)
      n168 = call "Main - Round Decimal Places.vi"("DecimalPlaces"=u8 0, "Number to round"=w324) -> ("Rounded number"=w323:dbl)  [unwired: 9 in]
      n169 = call "Main - Round Decimal Places.vi"("DecimalPlaces"=w312, "Number to round"=w331) -> ("Rounded number"=w330:dbl)  [unwired: 9 in]
      n170 = call "Main - Round Decimal Places.vi"("DecimalPlaces"=w312, "Number to round"=w329) -> ("Rounded number"=w328:dbl)  [unwired: 9 in]
      n171 = call "Main - Round Decimal Places.vi"("DecimalPlaces"=w312, "Number to round"=w314) -> ("Rounded number"=w327:dbl)  [unwired: 9 in]
      n172 = call "Main - Round Decimal Places.vi"("DecimalPlaces"=w312, "Number to round"=w326) -> ("Rounded number"=w325:dbl)  [unwired: 9 in]
      n173 = Bundle By Name(cluster=w353, "Calc.UCT.V Stress"=w330, "Calc.UCT.ALC"=w323, "Calc.UCT.H Change"=w328, "Calc.UCT.Deviator"=w327, "Calc.UCT.Axial Strain"=w325) -> (w354:T3)
      n174 = Build Array(w330, w323, w328, w327, w325) -> (w345:dbl[])
      n175 = for {
        tunnel: w345 -> [w359] mode=indexing
        tunnel: w320 -> [w358] mode=indexing
        tunnel: [w357] -> w344 mode=indexing
        n176 = Number To Fractional String(number=w359, precision (6)=w358) -> (F-format string=w357:string)  [unwired: 2 in]
      }
      n177 = Build Array (concatenate)(w321, w320) -> (w319:u8[])
      n178 = Build Array (concatenate)(w342, w345) -> (w341:dbl[])
      n179 = Build Array (concatenate)(w343, w344) -> (w340:string[])
    }
    frame "Shearbox" {
      w368 = u8 3 ("element")
      # "VL\nV Disp\nHL\nH Disp\nS Length Change\nShear Strain\nH Load Change\nNormal Stress\nShear Stress"
      n180 = Unbundle By Name(w389) -> ("Data.Diameter/Length"=w393:string, "Init.H Disp SB"=w391:sgl, "Init.H Load SB"=w386:sgl, "Data.Area"=w383:string, "Data.Height"=w366:string)
      n181 = Index Array(array=w379, index #1=3 ("index"), index #2=2 ("index"), index #3=0 ("index")) -> (element #1=w360:sgl, element #2=w362:sgl, element #3=w363:sgl)
      n182 = Fract/Exp String To Number(string=w393, default (0 dbl)=sgl 0.0 ("default (0 DBL)")) -> (number=w361:sgl)  [unwired: 2 in, 1 out]
      n183 = Fract/Exp String To Number(string=w366, default (0 dbl)=sgl 0.0 ("default (0 DBL)")) -> ()  [unwired: 2 in, 2 out]
      n184 = Fract/Exp String To Number(string=w383, default (0 dbl)=sgl 0.0 ("default (0 DBL)")) -> (number=w370:sgl)  [unwired: 2 in, 1 out]
      n185 = Subtract(x=w360, y=w391) -> (x-y=w376:sgl)
      n186 = Subtract(x=w362, y=w386) -> (x-y=w375:sgl)
      n187 = Divide(x=w376, y=w361) -> (x/y=w365:sgl)
      n188 = Multiply(x=w365, y=sgl 100.0) -> (x*y=w364:sgl)
      n189 = Divide(x=w363, y=w370) -> (x/y=w374:sgl)
      n190 = Multiply(x=w362, y=w370) -> (x*y=w369:sgl)
      n191 = Build Array(w368, w368, w368, w368, w368) -> (w380:u8[])
      n192 = Bundle By Name(cluster=w389, "Calc.SB.Speci LenC"=w376, "Calc.SB.Shear Strain"=w364, "Calc.SB.H LC"=w375, "Calc.SB.Normal Stress"=w374, "Calc.SB.Shear Stress"=w369) -> (w390:T3)
      n193 = Build Array(w376, w364, w375, w374, w369) -> (w382:sgl[])
      n194 = for {
        tunnel: w382 -> [w397] mode=indexing
        tunnel: w380 -> [w396] mode=indexing
        tunnel: [w395] -> w381 mode=indexing
        n195 = Number To Fractional String(number=w397, precision (6)=w396) -> (F-format string=w395:string)  [unwired: 2 in]
      }
      n196 = Build Array (concatenate)(w378, w380) -> (w371:u8[])
      n197 = Build Array (concatenate)(w379, w382) -> (w373:sgl[])
      n198 = Build Array (concatenate)(w377, w381) -> (w372:string[])
    }
  }
  n199 = disable-structure shown="Disabled" {
    frame Disabled {
      # "Area"
      n200 = Fract/Exp String To Number(default (0 dbl)=sgl 0.0 ("default (0 DBL)")) -> (number=w402:sgl)  [unwired: 3 in, 1 out]
      n201 = Divide(x=w402, y=sgl 2.0) -> (x/y=w404:sgl)
      n202 = Square(x=w404) -> (x^2=w405:sgl)
      n203 = Multiply(x=w405, y=3.141592653589793) -> (x*y=w403:dbl)
      n204 = Divide(x=w403, y=sgl 1000000.0) -> ()  [unwired: 1 out]
    }
    frame Enabled {
    }
  }
  n205 = Bundle By Name(cluster=w7, "Sensor Data"=w5, "Log Sensor"=w3, "1st Run"=FALSE, "Decimal"=w1) -> (→"DS out":T3)
  "error out" <- "error in (no error)"
